vi "CheeseRecive.vi"   [LabVIEW 2013]
uses:
  TCPServerStates.ctl
  VisionData.ctl
types:
  T1 = typedef "VisionData.ctl" = cluster{"Total":u8, "Timestamp":u32, "Horizontal":u8, "Vertical":u8, "Left Hot":bool, "Right Hot":bool}
  T2 = typedef "TCPServerStates.ctl" = enum16{"Listening", "Connected"}
  T3 = enum16{"Standard", "Buffered", "CRLF", "Immediate"}
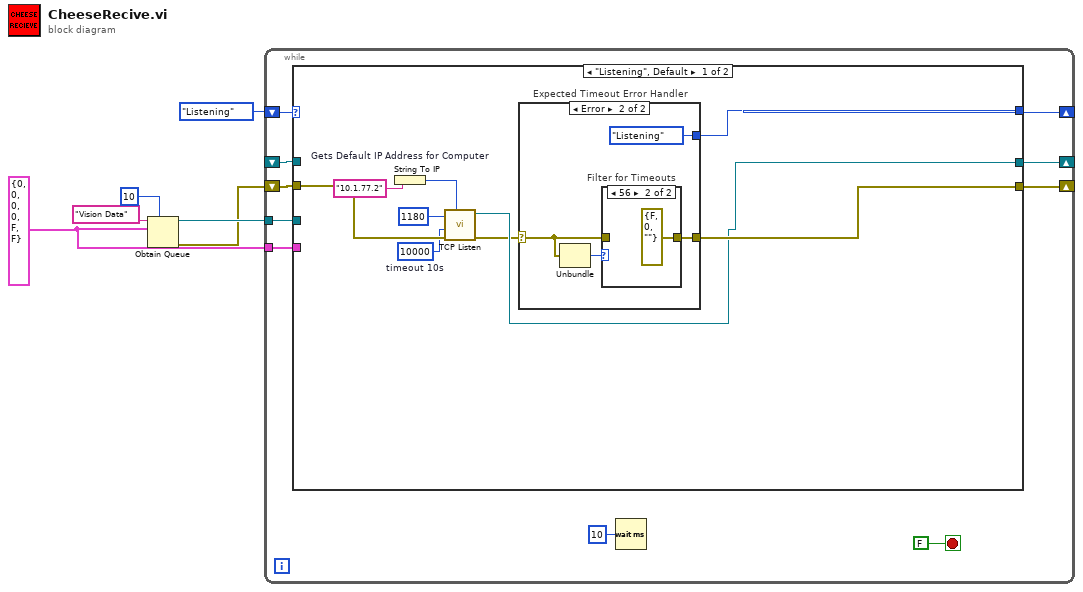
[diagram p0: block diagram]
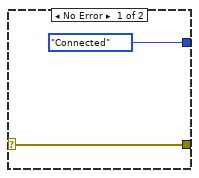
[diagram p2: hidden frame]
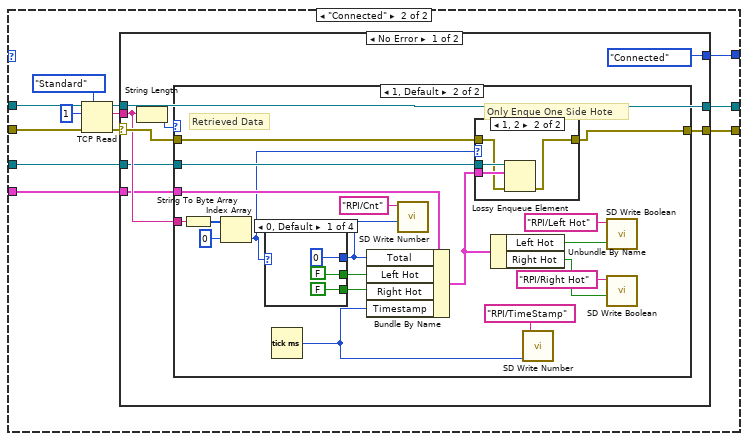
[diagram p4: hidden frame]
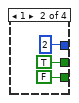
[diagram p7: hidden frame]
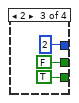
[diagram p8: hidden frame]
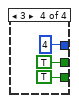
[diagram p9: hidden frame]
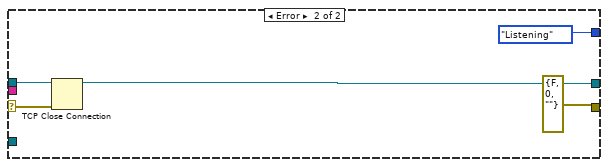
[diagram p10: hidden frame]
diagram:
  w1 = T1 {"Total"=0, "Timestamp"=0, "Horizontal"=0, "Vertical"=0, "Left Hot"=FALSE, "Right Hot"=FALSE}
  n1 = Obtain Queue(max queue size (-1, unlimited)=10, name (unnamed)="Vision Data", element data type=w1) -> (queue out=w3:refnum<queue>, error out=w2:errorcluster)  [unwired: 2 in, 1 out]
  n2 = while {
    shift-right: [w14] -> _
    shift-left: w2 -> [w12]
    shift-right: [w13] -> _
    shift-left: TCPServerStates."Listening" -> [w15]
    shift-right: [w11] -> _
    shift-left: _ -> [w10]
    tunnel: w3 -> [w9]
    tunnel: w1 -> [w8]
    stop <- FALSE stop-if-true
    n3 = case shown="\"Listening\", Default" w15 {
      tunnel: [w25 w42] -> w14
      tunnel: [w24 w41] -> w13
      tunnel: w12 -> [w23 w45]
      tunnel: [w22 w43] -> w11
      tunnel: w10 -> [_ w44]
      tunnel: w9 -> [_ w40]
      tunnel: w8 -> [_ w39]
      frame "Listening", Default {
        w21 = 10000  # timeout 10s
        n4 = String To IP "Gets Default IP Address for Computer"(1:"10.1.77.2" ("name")) -> (0:w18:u32)
        n5 = call <vilib>:"TCP Listen.vi"("net address"=w18, "error in (no error)"=w23, "timeout ms (wait forever: -1)"=w21, "port"=u16 1180) -> ("error out"=w19:errorcluster, "connection ID"=w22:refnum<k5>)  [unwired: 3 in, 3 out]
        n6 = case "Expected Timeout Error Handler" shown="Error" w19 {
          selector: w19 -> [w27 w29]
          tunnel: [w27 w30] -> w25
          tunnel: [TCPServerStates."Connected" TCPServerStates."Listening"] -> w24
          frame No Error {
          }
          frame Error {
            n7 = Unbundle(w29) -> ("code"=w31:i32)  [unwired: 2 out]
            n8 = case "Filter for Timeouts" shown="56" w31 {
              tunnel: [w32 errorcluster {"status"=FALSE, "code"=0, "source"=""} ("error constant")] -> w30
              tunnel: w29 -> [w32 _]
              frame 0, Default {
              }
              frame 56 {
              }
            }
          }
        }
      }
      frame "Connected" {
        n9 = TCP Read(connection ID=w44, bytes to read=1, error in (no error)=w45, 7:T3."Standard" ("mode (standard)")) -> (connection ID out=w35:refnum<k5>, data out=w37:string, error out=w36:errorcluster)  [unwired: 1 in]
        n10 = case shown="No Error" w36 {
          selector: w36 -> [w51 w91]
          tunnel: w37 -> [w48 _]
          tunnel: w35 -> [w52 w93]
          tunnel: [w52 w92] -> w43
          tunnel: [w50 errorcluster {"status"=FALSE, "code"=0, "source"=""} ("error IO")] -> w42
          tunnel: [TCPServerStates."Connected" TCPServerStates."Listening"] -> w41
          tunnel: w40 -> [w47 _]
          tunnel: w39 -> [w46 _]
          frame No Error {
            n11 = String Length(string=w48) -> (length=w53:i32)
            n12 = case shown="1, Default" w53 {
              tunnel: w51 -> [w54 w57]
              tunnel: [w54 w55] -> w50
              tunnel: w48 -> [_ w66]
              tunnel: w47 -> [_ w63]
              tunnel: w46 -> [_ w62]
              frame 0 {
                # "No Data"
              }
              frame 1, Default {
                # "Only Enque One Side Hote"
                # "Retrieved Data"
                n13 = String To Byte Array(string=w66) -> (unsigned byte array=w65:u8[])
                n14 = Index Array(array=w65, index=0) -> (element=w56:u8)
                n15 = case shown="0, Default" w56 {
                  tunnel: [u8 0 ("Total") u8 2 ("Total") u8 2 ("Total") u8 4 ("Total")] -> w59
                  tunnel: [FALSE ("Left Hot") TRUE ("Left Hot") FALSE ("Left Hot") TRUE ("Left Hot")] -> w60
                  tunnel: [FALSE ("Left Hot") FALSE ("Left Hot") TRUE ("Left Hot") TRUE ("Left Hot")] -> w61
                  frame 0, Default {
                  }
                  frame 1 {
                  }
                  frame 2 {
                  }
                  frame 3 {
                  }
                }
                n16 = Tick Count (ms)() -> (millisecond timer value=w71:u32)
                n17 = Bundle By Name(cluster=w62, "Total"=w59, "Left Hot"=w60, "Right Hot"=w61, "Timestamp"=w71) -> (w58:T1)
                n18 = call <vilib>:"SD Write Number.vi"("Numeric"=w59, "Name"="RPI/Cnt") -> ()  [unwired: 8 in, 2 out]
                n19 = case shown="1, 2" w56 {
                  tunnel: w63 -> [_ w78]
                  tunnel: w58 -> [_ w77]
                  tunnel: w57 -> [w74 w76]
                  tunnel: [w74 w75] -> w55
                  frame 0, Default {
                  }
                  frame 1, 2 {
                    n20 = Lossy Enqueue Element(queue=w78, element=w77, error in (no error)=w76) -> (error out=w75:errorcluster)  [unwired: 3 out]
                  }
                }
                n21 = Unbundle By Name(w58) -> ("Left Hot"=w70:bool, "Right Hot"=w69:bool)
                n22 = call <vilib>:"SD Write Number.vi"("Numeric"=w71, "Name"="RPI/TimeStamp") -> ()  [unwired: 8 in, 2 out]
                n23 = call <vilib>:"SD Write Boolean.vi"("Boolean"=w70, "Name"="RPI/Left Hot") -> ()  [unwired: 8 in, 2 out]
                n24 = call <vilib>:"SD Write Boolean.vi"("Boolean"=w69, "Name"="RPI/Right Hot") -> ()  [unwired: 8 in, 2 out]
              }
            }
          }
          frame Error {
            n25 = TCP Close Connection(connection ID=w93, error in (no error)=w91) -> (connection ID out=w92:refnum<k5>)  [unwired: 1 in, 1 out]
          }
        }
      }
    }
    n26 = Wait (ms)(milliseconds to wait=u32 10) -> ()  [unwired: 1 out]
  }
